vi "Global1.vi"() -> ()   [LabVIEW 2020]
panel:
  in  "产品型号":string
  in  "联机模式":enum16{"单机", "追溯"}(ring)
  out "用户信息":T1
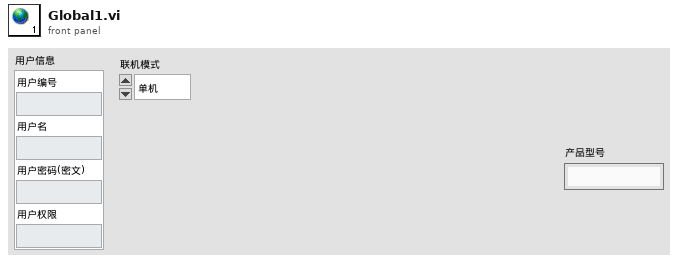
[diagram p1: front panel]
types:
  T1 = cluster{"用户编号":string, "用户名":string, "用户密码(密文)":string, "用户权限":string}
diagram:
